vi "Find COM Resources.vi"() -> (0 "Original list":string[](array[string]), 1 "COM only list":string[](array[string]))   [LabVIEW 2017, in "Vibratome.lvlib"]
uses:
  Vibratome/Vibratome.lvlib
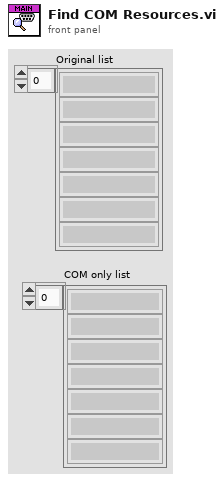
[diagram p1: front panel]
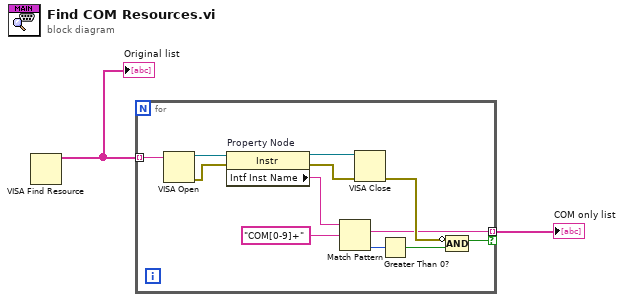
[diagram p0: block diagram]
diagram:
  n1 = VISA Find Resource() -> (3:w2:string[])  [unwired: 3 in, 2 out]
  "Original list" <- w2
  n2 = for {
    tunnel: w2 -> [w8] mode=indexing
    tunnel: [w3] -> w1 mode=indexing if=w4
    n3 = VISA Open(VISA resource name=w8) -> (VISA resource name=w14:refnum<visa-resource-name>, error out=w13:errorcluster)  [unwired: 4 in]
    n4 = property on="Property Node" class="Instr"(reference=w14, error in=w13) -> (reference out=w12:refnum<visa-resource-name>, error out=w11:errorcluster, "Intf Inst Name"=w10:string)
    n5 = Match Pattern(string=w10, regular expression="COM[0-9]+") -> (match substring=w3:string, offset past match=w7:i32)  [unwired: 1 in, 2 out]
    n6 = VISA Close(VISA resource name=w12, error in (no error)=w11) -> (error out=w6:errorcluster)
    n7 = Greater Than 0?(x=w7) -> (x > 0?=w5:bool)
    n8 = Compound Arithmetic op=AND(invert w6, w5) -> (w4:bool)
  }
  "COM only list" <- w1
